vi "NUMERIC OPERATIONS.vi"() -> ()   [LabVIEW 2019]
panel:
  out "QUOTIENT":dbl
  out "REMAINDER":dbl
  out "DIVISION":dbl
  out "MULTIPLICATION":dbl
  out "SUBRACTION":dbl
  out "ADDITION":dbl
  in  "NUMBER 2":dbl
  in  "NUMBER 1":dbl
  # "NUMERIC OPERATIONS"
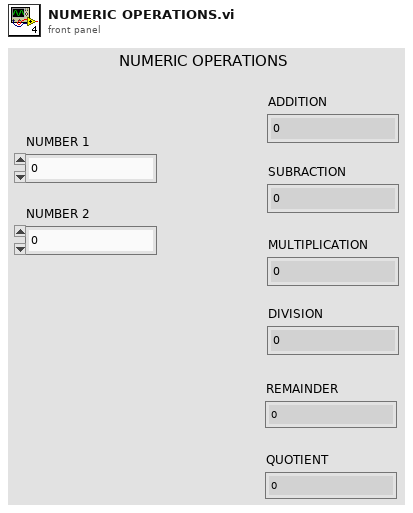
[diagram p1: front panel]
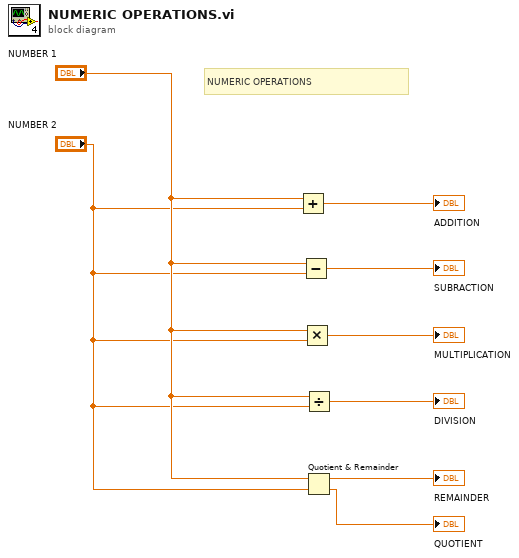
[diagram p0: block diagram]
diagram:
  # "NUMERIC OPERATIONS"
  n1 = Add(x="NUMBER 1", y="NUMBER 2") -> (x+y=→"ADDITION":dbl)
  n2 = Subtract(x="NUMBER 1", y="NUMBER 2") -> (x-y=→"SUBRACTION":dbl)
  n3 = Multiply(x="NUMBER 1", y="NUMBER 2") -> (x*y=→"MULTIPLICATION":dbl)
  n4 = Divide(x="NUMBER 1", y="NUMBER 2") -> (x/y=→"DIVISION":dbl)
  n5 = Quotient & Remainder(x="NUMBER 1", y="NUMBER 2") -> (x-y*floor(x/y)=→"REMAINDER":dbl, floor(x/y)=→"QUOTIENT":dbl)
